vi "Backpressure - no blocking.vi"(8 "error in (no error)":errorcluster) -> (0 "error out":errorcluster)   [LabVIEW 2026, in "Tests.lvlib"]
doc: "Update with test documentation"
uses:
  Tests.lvlib
  src/TypeDefs/Statement.ctl
  src/TypeDefs/Severity.ctl
  src/TypeDefs/DropPolicy.ctl
  <vilib>/addons/_JKI Toolkits/Caraya/classes/Assert/Assert True.vi
  <vilib>/addons/_JKI Toolkits/Caraya/classes/Test/Test.lvclass
  src/Lumberjack.lvlib
  <vilib>/addons/_JKI Toolkits/Caraya/classes/Assert/Assert.lvclass
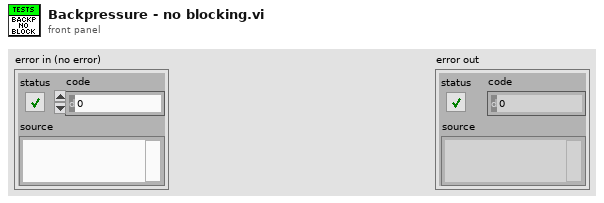
[diagram p1: front panel]
types:
  T1 = typedef "Lumberjack.lvlib/Statement.ctl" = cluster{"timestamp":timestamp, "level":T2, "sourceTag":string, "originVI":string, "message":string}
  T2 = typedef "Lumberjack.lvlib/Severity.ctl" = enum16{"OFF", "FATAL", "ERROR", "WARN", "INFO", "DEBUG", "TRACE", "ALL"}
  T3 = typedef "Lumberjack.lvlib/DropPolicy.ctl" = enum16{"DropOldest", "DropNewest", "LevelAware"}
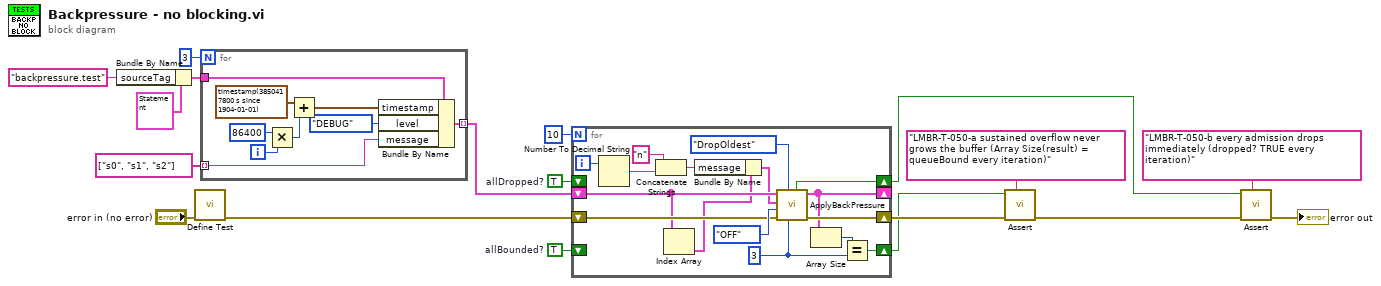
[diagram p0: block diagram]
diagram:
  w11 = TRUE  # allDropped?
  w12 = TRUE  # allBounded?
  n1 = Bundle By Name(cluster=T1 {"timestamp"=timestamp(0 s since 1904-01-01), "level"=enum."INFO", "sourceTag"="", "originVI"="", "message"=""} ("Statement"), "sourceTag"="backpressure.test") -> (w15:T1)
  n2 = call <vilib>:"Define Test.vi"("error in (no error)"="error in (no error)") -> ("error out"=w8:errorcluster)  [unwired: 9 in, 1 out]
  n3 = for {
    N: 3 -> [_]
    tunnel: w15 -> [w24]
    tunnel: string[] ["s0", "s1", "s2"] -> [w21] mode=indexing
    tunnel: [w20] -> w10 mode=indexing
    i -> [w22]
    n4 = Multiply(x=86400, y=w22) -> (x*y=w26:i32)
    n5 = Add(x=timestamp(3850417800 s since 1904-01-01), y=w26) -> (x+y=w23:timestamp)
    n6 = Bundle By Name(cluster=w24, "timestamp"=w23, "level"=Severity."DEBUG", "message"=w21) -> (w20:T1)
  }
  n7 = for {
    N: 10 -> [_]
    shift-right: [w38] -> _
    shift-left: w10 -> [w31]
    shift-right: [w34] -> w5
    shift-left: w12 -> [_]
    shift-right: [w37] -> w2
    shift-left: w11 -> [_]
    shift-right: [w40] -> w6
    shift-left: w8 -> [w39]
    i -> [w43]
    w35 = 3 ("queueBound")
    n8 = Number To Decimal String(number=w43) -> (decimal integer string=w32:string)  [unwired: 1 in]
    n9 = Concatenate Strings("n" ("string"), w32) -> (w29:string)
    n10 = Index Array(array=w31) -> (element=w28:T1)  [unwired: 1 in]
    n11 = Bundle By Name(cluster=w28, "message"=w29) -> (w30:T1)
    n12 = call "ApplyBackPressure.vi"("queueBound"=w35, "DropPolicy"=DropPolicy."DropOldest", "error in (no error)"=w39, "worstSeverityIn"=Severity."OFF", "incoming"=w30, "pending"=w31) -> ("error out"=w40:errorcluster, "result"=w38:T1[], "dropped"=w37:bool)  [unwired: 1 in, 2 out]
    n13 = Array Size(array=w38) -> (size(s)=w36:i32)
    n14 = Equal?(x=w36, y=w35) -> (x = y?=w34:bool)
  }
  n15 = call-poly <vilib>:"Assert.vi"("Label"="LMBR-T-050-a sustained overflow never grows the buffer (Array Size(result) = queueBound every iteration)" ("sourceTag"), "error in (no error)"=w6, "True?"=w5) -> ("error out"=w3:errorcluster)  [unwired: 7 in, 1 out]
  n16 = call-poly <vilib>:"Assert.vi"("Label"="LMBR-T-050-b every admission drops immediately (dropped? TRUE every iteration)" ("sourceTag"), "error in (no error)"=w3, "True?"=w2) -> ("error out"=→"error out":errorcluster)  [unwired: 7 in, 1 out]
